vi "Wait for Operation Complete.vi"(8 "error in (no error)":errorcluster, 9 "Maximum Time (10000ms)":u32=10000, 11 "VISA resource name":refnum<visa-resource-name>) -> (0 "error out":errorcluster, 3 "VISA resource name out":refnum<visa-resource-name>)   [LabVIEW 2017, in "Scope.lvlib" / "Tektronix DPO MSO 2000 4000 Series.lvlib"]
doc: "This VI waits for the instrument to complete the execution of all pending operations. The <B>Timeout</B> control specifies the maximum time to wait for operation complete in milliseconds."
uses:
  Tektronix DPO MSO 2000 4000 Series.lvlib
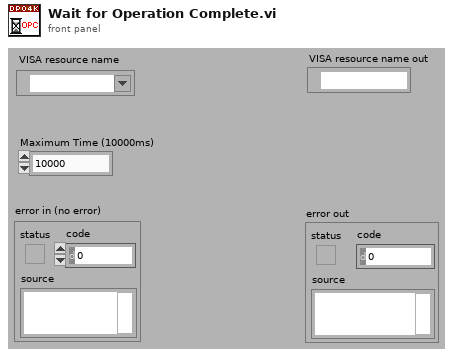
[diagram p1: front panel]
types:
  T1 = typedef "Scope.lvlib/Tektronix DPO MSO 2000 4000 Series.lvlib/Extended User Data.ctl" = cluster{"DPO MSO Series Model":u16}
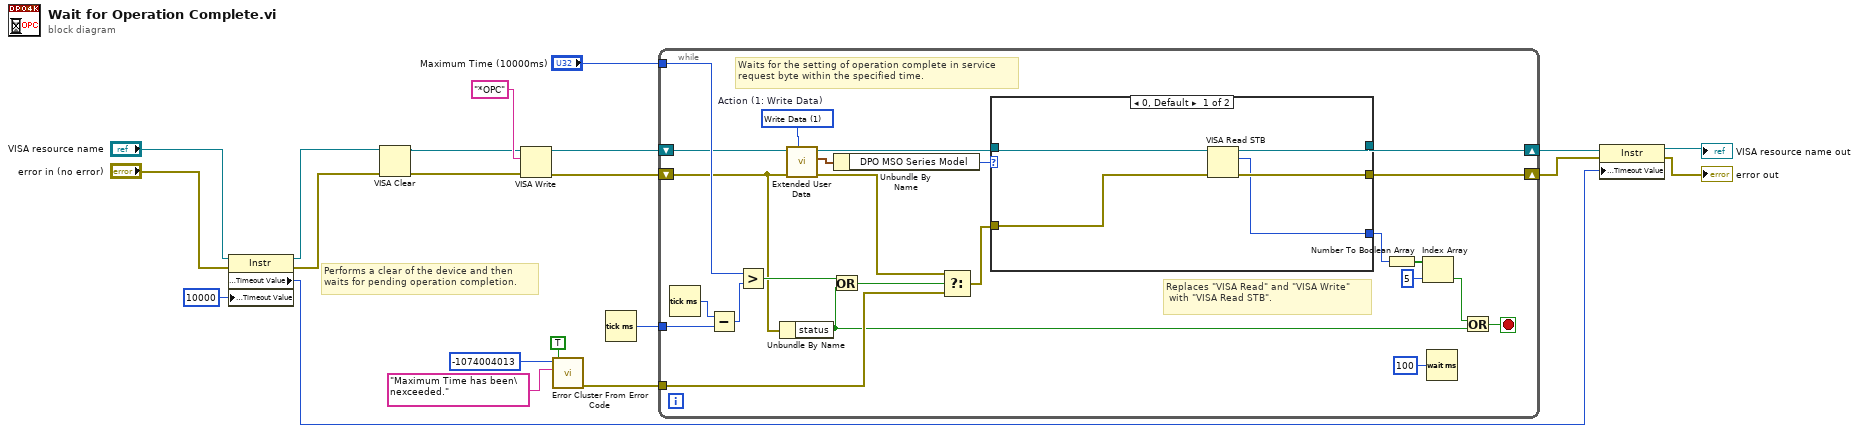
[diagram p0: block diagram]
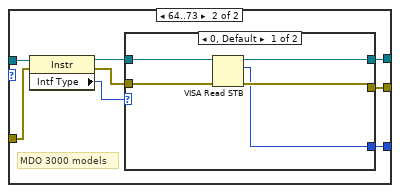
[diagram p2: hidden frame]
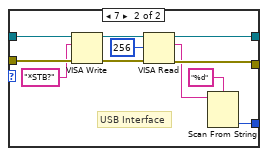
[diagram p3: hidden frame]
diagram:
  # "Performs a clear of the device and then\nwaits for pending operation completion."
  n1 = property class="Instr"(reference="VISA resource name", error in="error in (no error)", "General Settings:Timeout Value"=u32 10000) -> (reference out=w12:refnum<visa-resource-name>, error out=w11:errorcluster, "General Settings:Timeout Value"=w9:u32)
  n2 = VISA Clear(VISA resource name=w12, error in (no error)=w11) -> (VISA resource name out=w2:refnum<visa-resource-name>, error out=w1:errorcluster)
  n3 = VISA Write(VISA resource name=w2, write buffer="*OPC", error in (no error)=w1) -> (VISA resource name out=w18:refnum<visa-resource-name>, error out=w17:errorcluster)  [unwired: 1 out]
  n4 = call <vilib>:"Error Cluster From Error Code.vi"("show call chain? (False)"=TRUE, "error message (\"\")"="Maximum Time has been\nexceeded." ("error message (\"\")"), "error code (0)"=-1074004013) -> ("error out"=w16:errorcluster)  [unwired: 6 in]
  n5 = Tick Count (ms)() -> (millisecond timer value=w20:u32)
  n6 = while {
    tunnel: w20 -> [w42]
    tunnel: "Maximum Time (10000ms)" -> [w40]
    shift-right: [w31] -> w8
    shift-left: w18 -> [w26]
    shift-right: [w32] -> w7
    shift-left: w17 -> [w25]
    tunnel: w16 -> [w38]
    stop <- w37 stop-if-true
    w28 = 1 items=["Read Data", "Write Data", "Clear Data", "Clear ALL Data"]  # Action (1: Write Data)
    # "Replaces \"VISA Read\" and \"VISA Write\"\n with \"VISA Read STB\"."
    # "Waits for the setting of operation complete in service\nrequest byte within the specified time."
    n7 = Tick Count (ms)() -> (millisecond timer value=w43:u32)
    n8 = Subtract(x=w43, y=w42) -> (x-y=w41:u32)
    n9 = Greater?(x=w40, y=w41) -> (0:w35:bool)
    n10 = Unbundle By Name(w25) -> ("status"=w34:bool)
    n11 = call "Extended User Data.vi"("Action (1: Write Data)"=w28, "error in (no error)"=w25, "VISA resource name"=w26) -> ("error out"=w23:errorcluster, "User Data Out"=w27:T1, "VISA resource name out"=w24:refnum<visa-resource-name>)  [unwired: 6 in]
    n12 = Or(x=w35, y=w34) -> (x .or. y?=w39:bool)
    n13 = Unbundle By Name(w27) -> ("DPO MSO Series Model"=w22:u16)
    n14 = Select(t=w23, s=w39, f=w38) -> (s? t:f=w29:errorcluster)
    n15 = case shown="0, Default" w22 {
      tunnel: w24 -> [w50 w58]
      tunnel: [w49 w52] -> w32
      tunnel: [w48 w56] -> w31
      tunnel: [w47 w51] -> w30
      tunnel: w29 -> [w46 w57]
      frame 0, Default {
        n16 = VISA Read STB(8:w46, 11:w50) -> (0:w49:errorcluster, 2:w47:u16, 3:w48:refnum<visa-resource-name>)
      }
      frame 64..73 {
        # "MDO 3000 models"
        n17 = property class="Instr"(reference=w58, error in=w57) -> (reference out=w55:refnum<visa-resource-name>, error out=w53:errorcluster, "Intf Type"=w54:u16)
        n18 = case shown="0, Default" w54 {
          tunnel: [w61 w68] -> w56
          tunnel: w55 -> [w63 w74]
          tunnel: w53 -> [w62 w73]
          tunnel: [w60 w67] -> w52
          tunnel: [w59 w64] -> w51
          frame 0, Default {
            n19 = VISA Read STB(8:w62, 11:w63) -> (0:w60:errorcluster, 2:w59:u16, 3:w61:refnum<visa-resource-name>)
          }
          frame 7 {
            # "USB Interface"
            n20 = VISA Write(VISA resource name=w74, write buffer="*STB?", error in (no error)=w73) -> (VISA resource name out=w70:refnum<visa-resource-name>, error out=w71:errorcluster)  [unwired: 1 out]
            n21 = VISA Read(VISA resource name=w70, byte count=u32 256, error in (no error)=w71) -> (VISA resource name out=w68:refnum<visa-resource-name>, read buffer=w66:string, error out=w67:errorcluster)  [unwired: 1 out]
            n22 = Scan From String(format string="%d", input string=w66) -> (output 1=w64:i32)  [unwired: 3 in, 3 out]
          }
        }
      }
    }
    n23 = Number To Boolean Array(number=w30) -> (Boolean array=w45:bool[])
    n24 = Index Array(array=w45, index=5) -> (element=w36:bool)
    n25 = Wait (ms)(milliseconds to wait=u32 100) -> ()  [unwired: 1 out]
    n26 = Or(x=w36, y=w34) -> (x .or. y?=w37:bool)
  }
  n27 = property class="Instr"(reference=w8, error in=w7, "General Settings:Timeout Value"=w9) -> (reference out=→"VISA resource name out":refnum<visa-resource-name>, error out=→"error out":errorcluster)
